vi "GS Var Tool Common Ana User Settings.vi"(1 "Action(GET)":enum16{"GET", "SET"}(ring), 7 "Tool analog var User settigns in":T5[](array[typedef]) {"Scaling"."Offset" format="%.5f"; "Scaling"."Gain" format="%.5f"; "Limits and responces"."Limits"."H" format="%.3f"; "Limits and responces"."Limits"."L" format="%.3f"; "Limits and responces"."Limits"."HH" format="%.3f"; "Limits and responces"."Limits"."LL" format="%.3f"}, 9 "Tool digital var User settigns in":T1[](array[typedef]), 11 "error in (no error)":errorcluster) -> (8 "Tool Analog var User settigns out":T5[](array[typedef]) {"Scaling"."Offset" format="%.5f"; "Scaling"."Gain" format="%.5f"; "Limits and responces"."Limits"."H" format="%.3f"; "Limits and responces"."Limits"."L" format="%.3f"; "Limits and responces"."Limits"."HH" format="%.3f"; "Limits and responces"."Limits"."LL" format="%.3f"}, 10 "Tool digital var User settigns out":T1[](array[typedef]), 15 "error out":errorcluster)   [LabVIEW 2011]
uses:
  Measurments Handling/User Setting Analog Channel Bg.ctl
  Measurments Handling/Scaling.ctl
  Measurments Handling/Alarm Setup Analog.ctl
  Measurments Handling/Alarm Responce.ctl
  Measurments Handling/Action List.ctl
  Measurments Handling/Limits.ctl
  Measurments Handling/User Setting DigitalChannel.ctl
  Measurments Handling/Alarm Responce dig.ctl
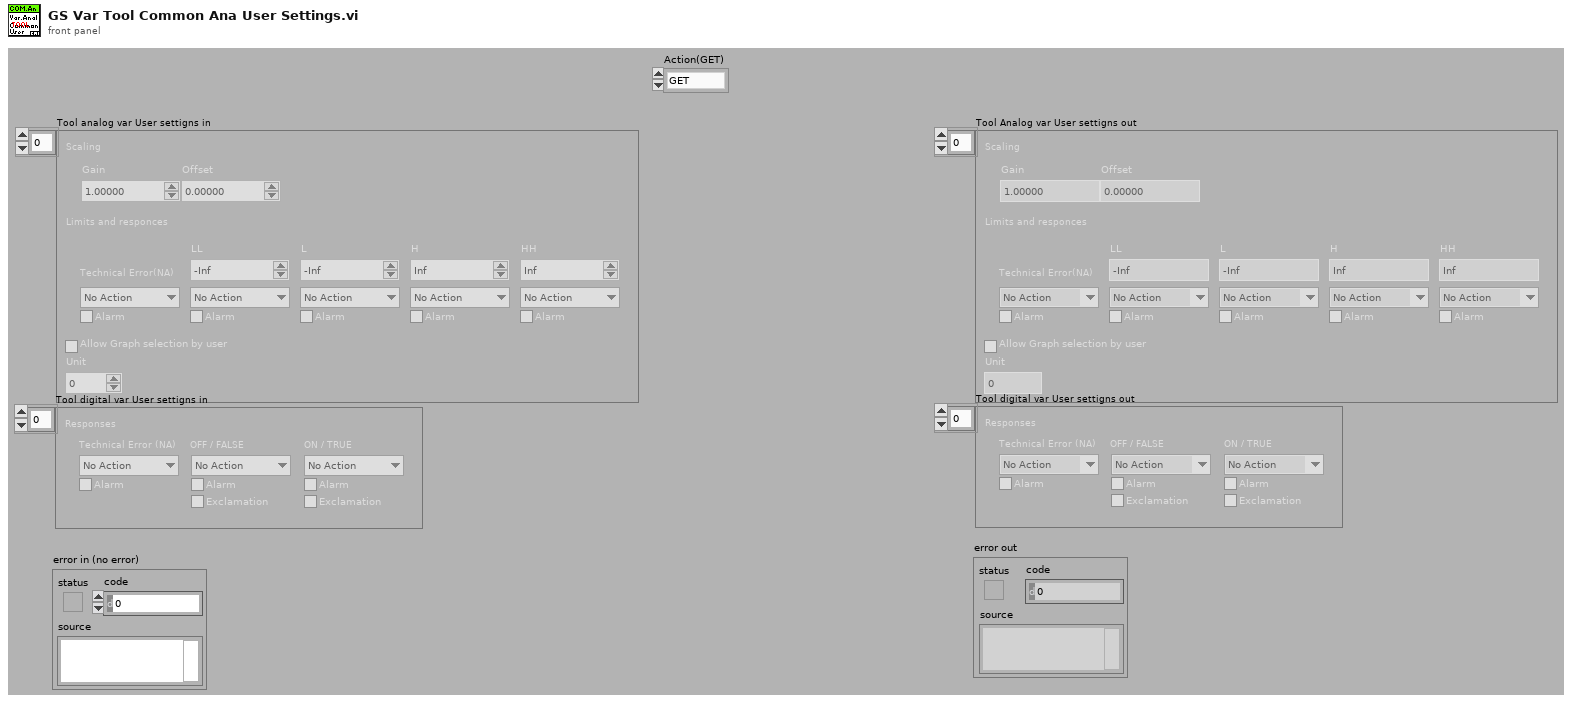
[diagram p1: front panel]
types:
  T1 = typedef "User Setting DigitalChannel.ctl" = cluster{"Responses":cluster{"Technical Error (NA)":T2, "OFF / FALSE":T4, "ON / TRUE":T4}}
  T2 = typedef "Alarm Responce.ctl" = cluster{"Action":T3, "Alarm":bool}
  T3 = typedef "Action List.ctl" = enum16{"No Action", "Stop Motor", "Turn Off HV"}
  T4 = typedef "Alarm Responce dig.ctl" = cluster{"Action":T3, "Alarm":bool, "Exclamation":bool}
  T5 = typedef "User Setting Analog Channel Bg.ctl" = cluster{"Scaling":T6, "Limits and responces":T7, "Allow Graph selection by user":bool, "Unit":u16}
  T6 = typedef "Scaling.ctl" = cluster{"Gain":dbl, "Offset":dbl}
  T7 = typedef "Alarm Setup Analog.ctl" = cluster{"Technical Error(NA)":T2, "LL":T2, "L":T2, "H":T2, "HH":T2, "Limits":T8}
  T8 = typedef "Limits.ctl" = cluster{"LL":dbl, "L":dbl, "H":dbl, "HH":dbl}
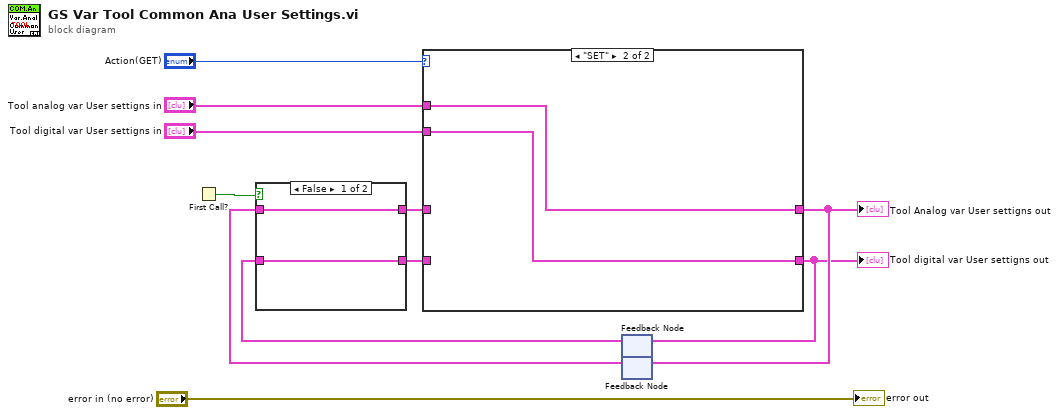
[diagram p0: block diagram]
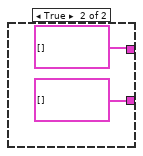
[diagram p2: hidden frame]
diagram:
  n1 = First Call?() -> (First Call?: T/F=w8:bool)
  n2 = feedback #1() -> (w2:T1[])  [unwired: 1 in]
  n3 = feedback #2() -> (w9:T5[])  [unwired: 1 in]
  n4 = case shown="False" w8 {
    tunnel: w9 -> [w13 _]
    tunnel: [w13 T5[] [] ("Common variables User settigns")] -> w6
    tunnel: [w12 T1[] [] ("Common variables User settigns")] -> w3
    tunnel: w2 -> [w12 _]
    frame False {
    }
    frame True {
    }
  }
  n5 = case shown="\"SET\"" "Action(GET)" {
    tunnel: [w17 w19] -> w7
    tunnel: w6 -> [w17 _]
    tunnel: "Tool analog var User settigns in" -> [_ w19]
    tunnel: [w16 w18] -> w4
    tunnel: w3 -> [w16 _]
    tunnel: "Tool digital var User settigns in" -> [_ w18]
    frame "GET", Default {
    }
    frame "SET" {
    }
  }
  "Tool Analog var User settigns out" <- w7
  "Tool digital var User settigns out" <- w4
  n6 = feedback-in #1(w4) -> ()
  n7 = feedback-in #2(w7) -> ()
  "error out" <- "error in (no error)"
